vi "meth.GetVariantWrapper.vi"(0 "class.GLue in":refnum<class "class.GLue.lvclass">, 11 "error in":errorcluster) -> (4 "class.GLue out":refnum<class "class.GLue.lvclass">, 8 "Variant":variant, 15 "error out":errorcluster)   [LabVIEW 2014, in "GLue.lvlib" / "class.GLue.lvclass"]
uses:
  class.GLue.lvclass
  class.GLue.lvclass/class.GLue.ctl
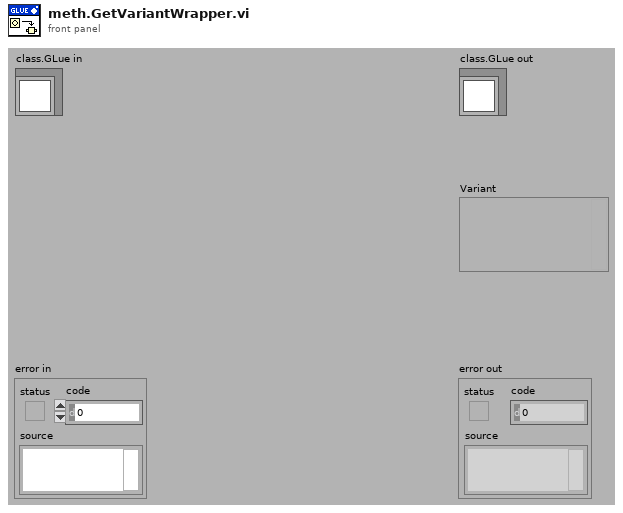
[diagram p1: front panel]
types:
  T1 = typedef "GLue.lvlib/class.GLue.lvclass/typedef.Types.ctl" = enum16{"Nil", "Bool", "LightUserData", "Number", "String", "Table", "Function", "UserData", "Thread"}
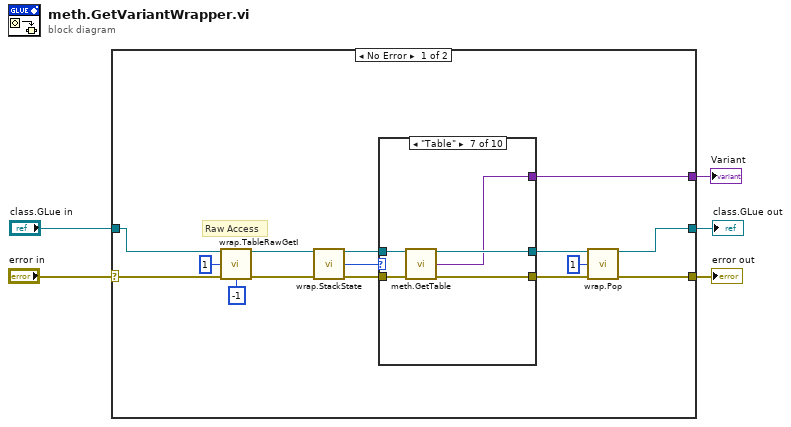
[diagram p0: block diagram]
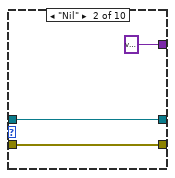
[diagram p3: hidden frame]
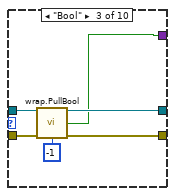
[diagram p4: hidden frame]
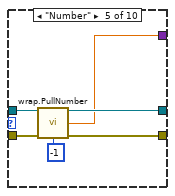
[diagram p6: hidden frame]
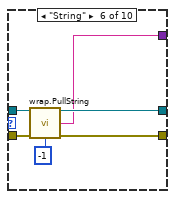
[diagram p7: hidden frame]
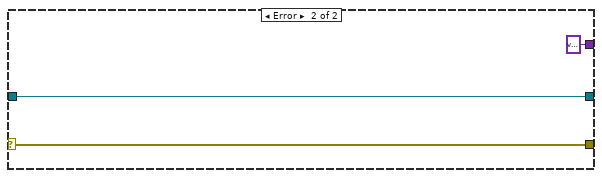
[diagram p11: hidden frame]
diagram:
  n1 = case shown="No Error" "error in" {
    selector: "error in" -> [w8 w59]
    tunnel: [w19 w59] -> w4
    tunnel: [w20 w58] -> w2
    tunnel: "class.GLue in" -> [w9 w58]
    tunnel: [w18 variant ("Cluster")] -> w1
    frame No Error {
      # "Raw Access"
      n2 = call "wrap.TableRawGetI.vi"("class.GLue in"=w9, "n"=1, "error in (no error)"=w8, "Index"=-1) -> ("class.GLue out"=w7:refnum<class "class.GLue.lvclass">, "error out"=w6:errorcluster)  [unwired: 10 in]
      n3 = call "wrap.StackState.vi"("class.GLue in"=w7, "error in (no error)"=w6) -> ("class.GLue out"=w16:refnum<class "class.GLue.lvclass">, "TopType"=w17:T1, "error out"=w15:errorcluster)  [unwired: 10 in, 1 out]
      n4 = case shown="\"Table\"" w17 {
        tunnel: w16 -> [w21 w25 w31 w33 w39 w45 w50 w52 w54 w56]
        tunnel: w15 -> [w22 w24 w30 w32 w38 w44 w49 w51 w53 w55]
        tunnel: [w22 w24 w28 w32 w36 w42 w46 w51 w53 w55] -> w14
        tunnel: [w21 w25 w27 w33 w37 w43 w48 w52 w54 w56] -> w13
        tunnel: [_ variant ("variant") w26 _ w34 w41 w47 _ _ _] -> w18
        frame Default {
        }
        frame "Nil" {
        }
        frame "Bool" {
          n5 = call "wrap.PullBool.vi"("class.GLue in"=w31, "error in (no error)"=w30, "Index"=-1) -> ("class.GLue out"=w27:refnum<class "class.GLue.lvclass">, "Boolean"=w26:bool, "error out"=w28:errorcluster)  [unwired: 10 in]
        }
        frame "LightUserData" {
        }
        frame "Number" {
          n6 = call "wrap.PullNumber.vi"("class.GLue in"=w39, "error in (no error)"=w38, "Index"=-1) -> ("class.GLue out"=w37:refnum<class "class.GLue.lvclass">, "Number"=w34:dbl, "error out"=w36:errorcluster)  [unwired: 10 in]
        }
        frame "String" {
          n7 = call "wrap.PullString.vi"("class.GLue in"=w45, "error in (no error)"=w44, "Index"=-1) -> ("class.GLue out"=w43:refnum<class "class.GLue.lvclass">, "String"=w41:string, "error out"=w42:errorcluster)  [unwired: 10 in]
        }
        frame "Table" {
          n8 = call "meth.GetTable.vi"("class.GLue in"=w50, "error in (no error)"=w49) -> ("class.GLue out"=w48:refnum<class "class.GLue.lvclass">, "Table"=w47:variant, "error out"=w46:errorcluster)  [unwired: 11 in]
        }
        frame "Function" {
        }
        frame "UserData" {
        }
        frame "Thread" {
        }
      }
      n9 = call "wrap.Pop.vi"("class.GLue in"=w13, "Num"=1, "error in (no error)"=w14) -> ("class.GLue out"=w20:refnum<class "class.GLue.lvclass">, "error out"=w19:errorcluster)  [unwired: 11 in]
    }
    frame Error {
    }
  }
  "error out" <- w4
  "class.GLue out" <- w2
  "Variant" <- w1
